vi "Configure Modulation (Frequency).vi"(0 "VISA resource name":refnum<visa-resource-name>, 1 "Enable Frequency Modulation (T: Enable)":bool=TRUE, 2 "File Path":string, 5 "Channel (0: Channel 1)":u16(ring) items=["Channel 1", "Channel 2"], 7 "FM Source (0: Internal)":u16(ring) items=["Internal", "External"], 9 "Modulation Waveform (0: Sine)":u16(ring) items=["Sine", "Square", "Triangle", "Ramp", "Down Ramp", "Noise", "User 1", "User 2", "User 3", "User 4", "Edit Memory", "Edit Path"], 11 "error in (no error)":errorcluster, 12 "Modulation Frequency (100.00 Hz)":dbl=100.0, 13 "Peak Deviation (100.00 Hz)":dbl=100.0) -> (4 "VISA resource name out":refnum<visa-resource-name>, 15 "error out":errorcluster)   [LabVIEW 2015, in "Tektronix AFG 3000 Series.lvlib"]
doc: "Configures and enables frequency modulation (FM). In FM, the frequency of the carrier is varied by the frequency of the modulating waveform."
uses:
  Tektronix AFG 3000 Series.lvlib
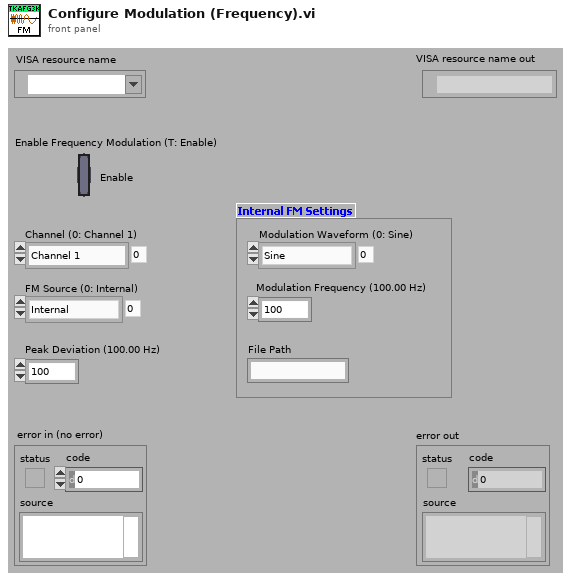
[diagram p1: front panel]
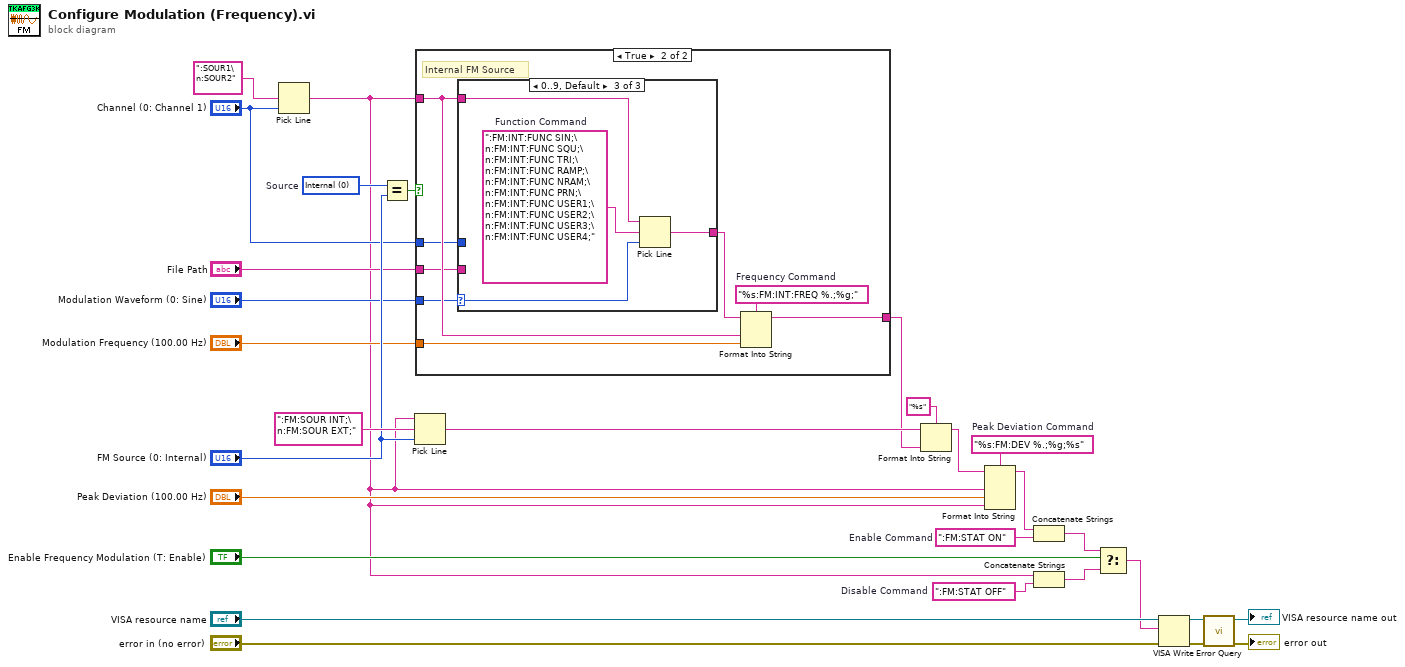
[diagram p0: block diagram]
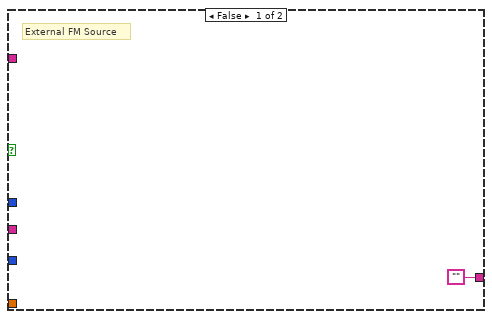
[diagram p2: hidden frame]
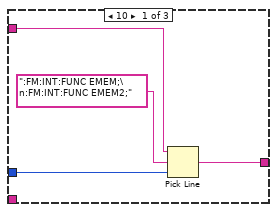
[diagram p3: hidden frame]
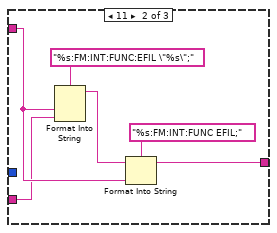
[diagram p4: hidden frame]
diagram:
  w20 = ":FM:STAT ON"  # Enable Command
  w10 = u16 0 items=["Internal", "External"]  # Source
  w23 = "%s:FM:DEV %.;%g;%s"  # Peak Deviation Command
  w18 = ":FM:STAT OFF"  # Disable Command
  n1 = Pick Line(multi-line string=":SOUR1\n:SOUR2" ("string (\"\")"), line index="Channel (0: Channel 1)") -> (output string=w1:string)  [unwired: 1 in]
  n2 = Equal?(x=w10, y="FM Source (0: Internal)") -> (x = y?=w12:bool)
  n3 = Pick Line(string ("")=w1, multi-line string=":FM:SOUR INT;\n:FM:SOUR EXT;" ("Source Command"), line index="FM Source (0: Internal)") -> (output string=w8:string)
  n4 = case shown="True" w12 {
    tunnel: ["" w37] -> w7
    tunnel: w1 -> [_ w35]
    tunnel: "Modulation Waveform (0: Sine)" -> [_ w34]
    tunnel: "Modulation Frequency (100.00 Hz)" -> [_ w36]
    tunnel: "File Path" -> [_ w32]
    tunnel: "Channel (0: Channel 1)" -> [_ w31]
    frame False {
      # "External FM Source"
    }
    frame True {
      w38 = "%s:FM:INT:FREQ %.;%g;"  # Frequency Command
      # "Internal FM Source"
      n5 = case shown="0..9, Default" w34 {
        selector: w34 -> [_ _ w51]
        tunnel: [w41 w45 w50] -> w33
        tunnel: w35 -> [w39 w44 w49]
        tunnel: w32 -> [_ w43 _]
        tunnel: w31 -> [w40 _ _]
        frame 10 {
          n6 = Pick Line(string ("")=w39, multi-line string=":FM:INT:FUNC EMEM;\n:FM:INT:FUNC EMEM2;", line index=w40) -> (output string=w41:string)
        }
        frame 11 {
          n7 = Format Into String(format string="%s:FM:INT:FUNC:EFIL \"%s\";", w44, w43) -> (resulting string=w48:string)  [unwired: 2 in, 1 out]
          n8 = Format Into String(format string="%s:FM:INT:FUNC EFIL;", initial string=w48, w44) -> (resulting string=w45:string)  [unwired: 1 in, 1 out]
        }
        frame 0..9, Default {
          w52 = ":FM:INT:FUNC SIN;\n:FM:INT:FUNC SQU;\n:FM:INT:FUNC TRI;\n:FM:INT:FUNC RAMP;\n:FM:INT:FUNC NRAM;\n:FM:INT:FUNC PRN;\n:FM:INT:FUNC USER1;\n:FM:INT:FUNC USER2;\n:FM:INT:FUNC USER3;\n:FM:INT:FUNC USER4;"  # Function Command
          n9 = Pick Line(string ("")=w49, multi-line string=w52, line index=w51) -> (output string=w50:string)
        }
      }
      n10 = Format Into String(format string=w38, initial string=w33, w35, w36) -> (resulting string=w37:string)  [unwired: 1 in, 1 out]
    }
  }
  n11 = Format Into String(format string="%s", initial string=w8, w7) -> (resulting string=w6:string)  [unwired: 1 in, 1 out]
  n12 = Format Into String(format string=w23, initial string=w6, w1, "Peak Deviation (100.00 Hz)", w1) -> (resulting string=w21:string)  [unwired: 1 in, 1 out]
  n13 = Concatenate Strings(w21, w20) -> (w14:string)
  n14 = Concatenate Strings(w1, w18) -> (w16:string)
  n15 = Select(t=w14, s="Enable Frequency Modulation (T: Enable)", f=w16) -> (s? t:f=w15:string)
  n16 = VISA Write(VISA resource name="VISA resource name", write buffer=w15, error in (no error)="error in (no error)") -> (VISA resource name out=w26:refnum<visa-resource-name>, error out=w27:errorcluster)  [unwired: 1 out]
  n17 = call "Error Query.vi"("error in (no error)"=w27, "VISA resource name"=w26) -> ("error out"=→"error out":errorcluster, "VISA resource name out"=→"VISA resource name out":refnum<visa-resource-name>)  [unwired: 6 in, 2 out]
